vi "RunAcquisition.vi"(8 "error in (no error)":errorcluster, 11 "ScopePluginsBase in":refnum<class "ScopePluginsBase.lvclass">) -> (0 "error out":errorcluster, 2 "Waveforms":T1[](array[typedef]), 3 "ScopePluginsBase out":refnum<class "ScopePluginsBase.lvclass">)   [LabVIEW 2018, in "ScopePlugins.lvlib" / "ScopePluginsBase.lvclass"]
uses:
  ScopePluginsBase.lvclass
  ScopeShared/Waveform.ctl
  <userlib>/NIST/BaseClasses/Object_class/BaseObject.lvclass
  ScopeShared/ScopeShared.lvlib
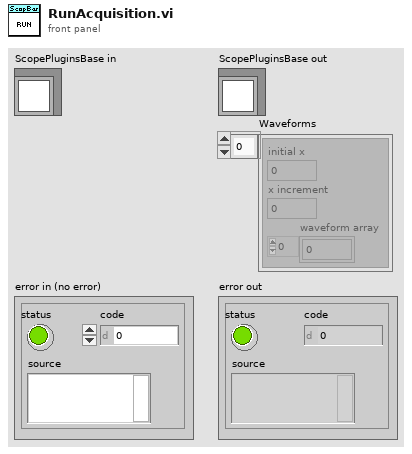
[diagram p1: front panel]
types:
  T1 = typedef "ScopeShared.lvlib/Waveform.ctl" = cluster{"initial x":dbl, "x increment":dbl, "waveform array":dbl[]}
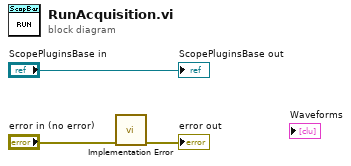
[diagram p0: block diagram]
diagram:
  n1 = call <userlib>:"Implementation Error.vi"("error in (no error)"="error in (no error)") -> ("error out"=→"error out":errorcluster)  [unwired: 10 in]
  "ScopePluginsBase out" <- "ScopePluginsBase in"
